vi "WriteB.vi"(0 "val":u8, 1 "offset":u32) -> ()   [LabVIEW 2015]
uses:
  ESLSCDLL.dll
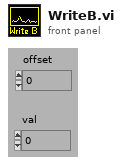
[diagram p1: front panel]
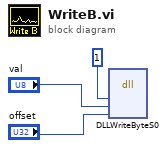
[diagram p0: block diagram]
diagram:
  n1 = dll-call lib="C:/ENTW/PCIE/64bit/lv64/1cam/board.vis/ESLSCDLL.dll" fn="DLLWriteByteS0"("drv"=u32 1, "DataByte"="val", "PortOff"="offset") -> ()  [unwired: 7 in, 2 out]
